vi "TakeHostControl.vi"(8 "error in (no error)":errorcluster, 11 "SM1000-control in":T1) -> (0 "error out":errorcluster, 3 "SM1000-control out":T1)   [LabVIEW 2013, in "HardwareCharacterization.lvlib" / "HC-SM1000.lvclass"]
doc: "Requests exclusive control of the EC1000.\n\nExclusive control will not be granted if the EC1000 is currently executing a job. Use the 'GetJobStatus' command to determine if the EC1000 is in a proper state before issuing this command.\n\nCommand: \"TakeHostControl\" or 2\nReturns: \"0\""
uses:
  HC-SM1000.lvclass
  Object-reference.ctl
  HC-SM1000.lvclass/HC-SM1000.ctl
  Custom-errors.ctl
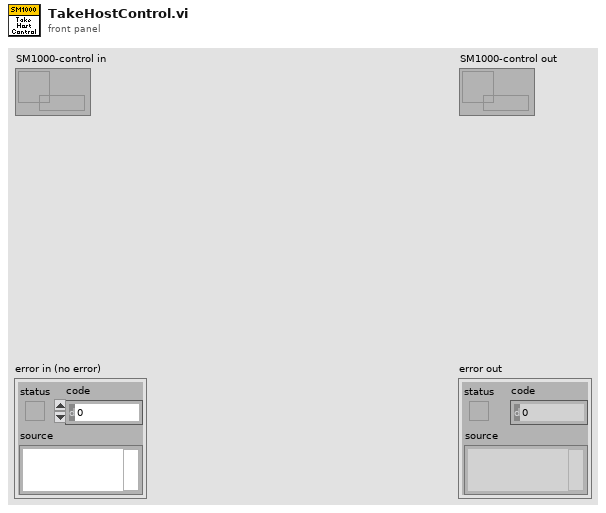
[diagram p1: front panel]
types:
  T1 = typedef "HardwareCharacterization.lvlib/HC-SM1000.lvclass/Object-reference.ctl" = refnum<data-value>
  T2 = typedef "HardwareCharacterization.lvlib/HC-SM1000.lvclass/Custom-errors.ctl" = enum16{"No error", "Not implemented", "Command not recognized", "Invalid input", "No connection", "Timeout", "Resource not loaded"}
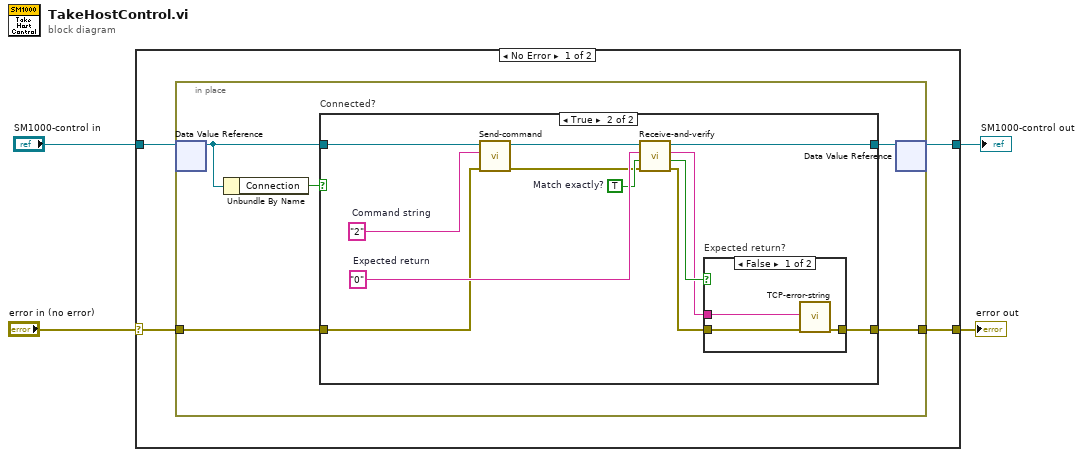
[diagram p0: block diagram]
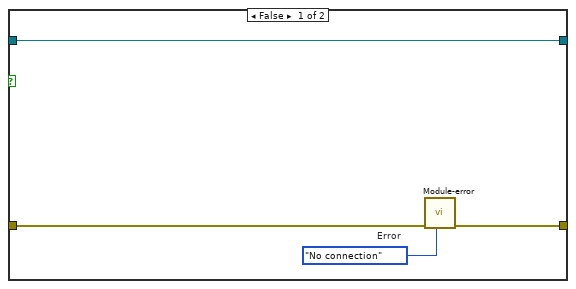
[diagram p2: hidden frame]
diagram:
  n1 = case shown="No Error" "error in (no error)" {
    selector: "error in (no error)" -> [w6 w35]
    tunnel: [w5 w35] -> w3
    tunnel: [w7 w34] -> w1
    tunnel: "SM1000-control in" -> [w8 w34]
    frame No Error {
      n2 = in-place {
        in-place-border: w6 -> [w13]
        in-place-border: [w10] -> w5
        n3 = in-place-dvr #1(w8) -> (w11:refnum<class "HC-SM1000.lvclass">)  [unwired: 1 out]
        n4 = Unbundle By Name(w11) -> ("Connection"=w12:bool)
        n5 = case "Connected?" shown="True" w12 {
          tunnel: w13 -> [w17 w21]
          tunnel: w11 -> [w15 w29]
          tunnel: [w16 w19] -> w10
          tunnel: [w15 w18] -> w9
          frame False {
            w14 = Custom-errors."No connection"  # Error
            n6 = call "Module-error.vi"("Error"=w14, "error in (no error)"=w17) -> ("error out"=w16:errorcluster)  [unwired: 9 in]
          }
          frame True {
            w25 = TRUE  # Match exactly?
            w26 = "0"  # Expected return
            w27 = "2"  # Command string
            n7 = call "Send-command.vi"("error in (no error)"=w21, "Command string"=w27, "SM1000-control in"=w29) -> ("error out"=w24:errorcluster, "SM1000-control out"=w28:refnum<class "HC-SM1000.lvclass">)  [unwired: 7 in]
            n8 = call "Receive-and-verify.vi"("error in (no error)"=w24, "Match exactly?"=w25, "Expected return string"=w26, "SM1000-control in"=w28) -> ("error out"=w20:errorcluster, "Verified?"=w23:bool, "Return string"=w22:string, "SM1000-control out"=w18:refnum<class "HC-SM1000.lvclass">)  [unwired: 4 in]
            n9 = case "Expected return?" shown="False" w23 {
              tunnel: w22 -> [w32 _]
              tunnel: w20 -> [w31 w33]
              tunnel: [w30 w33] -> w19
              frame False {
                n10 = call "TCP-error-string.vi"("error in (no error)"=w31, "Retun code"=w32) -> ("error out"=w30:errorcluster)  [unwired: 9 in]
              }
              frame True {
              }
            }
          }
        }
        n11 = in-place-dvr #1(w9) -> (w7:T1)  [unwired: 1 out]
      }
    }
    frame Error {
    }
  }
  "error out" <- w3
  "SM1000-control out" <- w1
